vi "SetOutputState.vi"(8 "error in (no error)":errorcluster caption="entrée d'erreur (pas d'erreur)", 10 "Output State":bool, 11 "Water Level en entrée":refnum<class "Water Level.lvclass">) -> (0 "error out":errorcluster caption="sortie d'erreur", 3 "Water Level en sortie":refnum<class "Water Level.lvclass">)   [LabVIEW 2015, in "Water Level.lvclass"]
uses:
  Water Level.lvclass
  Simulation/Simulation Data_Global.vi
  Simulation/Simulation.lvlib
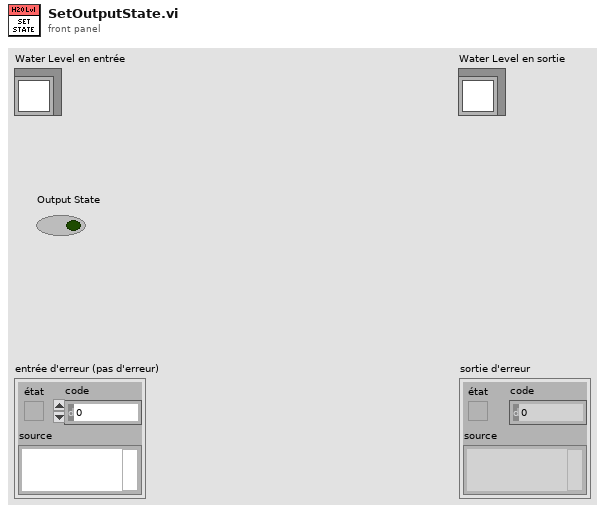
[diagram p1: front panel]
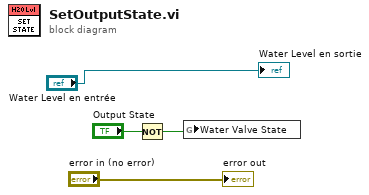
[diagram p0: block diagram]
diagram:
  n1 = Not(x="Output State") -> (.not. x?=w3:bool)
  n2 = global write "Simulation Data_Global.vi" "Water Valve State"(w3) -> ()
  "error out" <- "error in (no error)"
  "Water Level en sortie" <- "Water Level en entrée"
